vi "Filter.vi"(8 "error in (no error)":errorcluster, 10 "Test Suite":refnum<class "LUnit Test Suite.lvclass">, 11 "Static Filter in":refnum<class "Static Filter.lvclass">) -> (0 "error out":errorcluster, 2 "Filtered Test Suite":refnum<class "LUnit Test Suite.lvclass">)   [LabVIEW 2020, in "Static Filter.lvclass"]
uses:
  Static Filter.lvclass
  API/LUnit Test Suite/LUnit Test Suite.lvclass
  Static Filter.lvclass/Static Filter.ctl
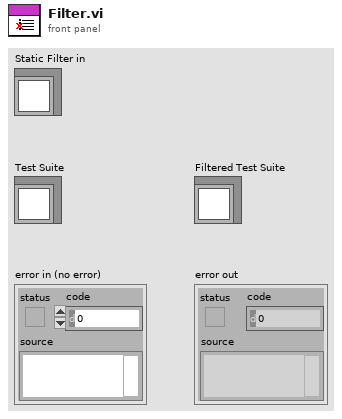
[diagram p1: front panel]
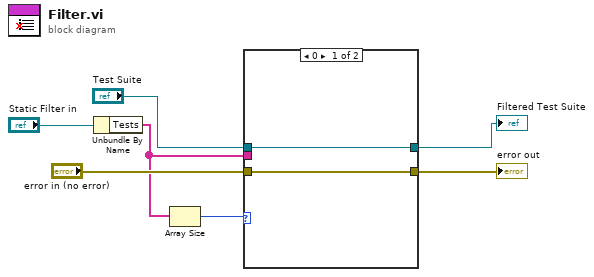
[diagram p0: block diagram]
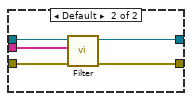
[diagram p2: hidden frame]
diagram:
  n1 = Unbundle By Name("Static Filter in") -> ("Tests"=w2:string[])
  n2 = Array Size(array=w2) -> (size(s)=w1:i32)
  n3 = case shown="0" w1 {
    tunnel: "error in (no error)" -> [w8 w14]
    tunnel: [w8 w13] -> w6
    tunnel: "Test Suite" -> [w9 w12]
    tunnel: [w9 w11] -> w4
    tunnel: w2 -> [_ w10]
    frame 0 {
    }
    frame Default {
      n4 = call "Filter.vi"("error in (no error)"=w14, "Selected Runnables"=w10, "LUnit Test Suite In"=w12) -> ("error out"=w13:errorcluster, "LUnit Test Suite Out"=w11:refnum<class "LUnit Test Suite.lvclass">)  [unwired: 7 in]
    }
  }
  "error out" <- w6
  "Filtered Test Suite" <- w4
